vi "Perform Measurement.vi"(7 "error in (no error)":errorcluster, 8 "Measure Call Context in":refnum<class "Measure Call Context.lvclass">, 10 "measurement configuration":T2={"Mode of operation"=enum."Power on the DUT", "Source enable/disable"=FALSE, "Load enable/disable"=FALSE, "Source resource names"=[], "Load resource names"=[], "Power ON/Source system configuration"=enum."Series", "Power ON/Source output function"=0, "Source sweep scale"="", "Power ON V/I Source start level"=0.0, "Source stop level"=0.0, "Source sweep points/points per decade"=0, "Source voltage/current level range"=0.0, "Power ON/Source sense"=0, "Source limit symmetry"=enum."Symmetric", "Power ON/Source current/voltage limit range"=0.0, "Source current/voltage limit low"=0.0, "Source current/voltage limit high"=0.0, "Source source delay"=0.0, "Source aperture time"=0.0, "Source transient response"=0, "Source voltage/current gain bandwidth"=0.0, "Source voltage/current compensation frequency"=0.0, "Source voltage/current pole-zero ratio"=0.0, "Load system configuration"=enum."Series", "Load output function"=0, "Load device voltage/current rating"=50.0, "Load sweep scale"="", "Load start level"=0.0, "Load stop level"=0.0, "Load sweep points/points per decade"=0, "Load voltage/current level range"=0.0, "Load sense"=0, "Load limit symmetry"=enum."Symmetric", "Load current/voltage limit range"=0.0, "Load current/voltage limit low"=0.0, "Load current/voltage limit high"=0.0, "Load source delay"=0.0, "Load aperture time"=0.0, "Load transient response"=0, "Load voltage/current gain bandwidth"=0.0, "Load voltage/current compensation frequency"=0.0, "Load voltage/current pole-zero ratio"=0.0, "Load source trigger"="", "Load measure trigger"="", "Measurement timeout"=10.0} {"Measurement timeout" format="%.3p"; "Load device voltage/current rating" format="%#_6pA"; "Load output function" items=["DC Voltage"=1006, "DC Current"=1007, "Pulse Voltage"=1049, "Pulse Current"=1050]; "Power ON/Source output function" items=["DC Voltage"=1006, "DC Current"=1007, "Pulse Voltage"=1049, "Pulse Current"=1050]; "Load sweep points/points per decade" format="%#_6p"; "Power ON V/I Source start level" format="%#_6p"; "Load sense" items=["Symmetric", "Asymmetric"]; "Load transient response" items=["Slow"=1041, "Normal"=1038, "Fast"=1039, "Custom"=1042]; "Power ON/Source sense" items=["Local"=1008, "Remote"=1009]; "Source transient response" items=["Slow"=1041, "Normal"=1038, "Fast"=1039, "Custom"=1042]; "Load current/voltage limit low" format="%#_6p"; "Load current/voltage limit range" format="%#_6p"; "Load voltage/current level range" format="%#_6p"; "Source current/voltage limit high" format="%#_6p"; "Source current/voltage limit low" format="%#_6p"; "Power ON/Source current/voltage limit range" format="%#_6p"; "Source voltage/current level range" format="%#_6p"}) -> (0 "error out":errorcluster, 1 "Measure Call Context out":refnum<class "Measure Call Context.lvclass">, 3 "Measurement Results":T1)   [LabVIEW 2021, in "Sweep_Channel Ganging.lvlib"]
doc: "This VI Perform different API calls to do Sweep Measurement in different configurations of Source and Load like \n\nSingle-Ganged \nGanged-Ganged\nGanged-Single\nSingle-Single"
uses:
  Sweep_Channel Ganging.lvlib
  shared subVIs/ctl/NIDCPower_channel_ganging - ctl - ganged config.ctl
  shared subVIs/ctl/NIDCPower_channel_ganging - ctl - channel mode.ctl
  shared/Single/controls/Initialize Resource Config-Single.ctl
  shared/Ganging/controls/Initialize Resource Config-Ganging.ctl
  shared subVIs/ctl/NIDCPower_channel_ganging - ctl - ganged session.ctl
  <instrlib>/niDCPower/nidcpower.llb/niDCPower Wait For Event - Event.ctl
  Measurement Results.ctl
  ctl/Sweep fetch measurement control.ctl
  shared/Single/controls/Source to Sequence Config-Single.ctl
  shared/Ganging/controls/Source to Sequence Config-Ganging.ctl
  shared/Single/controls/Load to Sequence Config-Single.ctl
  shared/Ganging/controls/Load to Sequence Config-Ganging.ctl
  shared/Common/controls/Start and Wait for Event.ctl
  shared/Ganging/controls/Abort Single Point-Ganging.ctl
  shared/Single/controls/Abort Single Point-Single.ctl
  ctl/Sweep perform meaasurement.ctl
  <vilib>/Plug-In SDKs/Measurements/Measure Call Context/Measure Call Context.lvclass
  Measurement Configuration.ctl
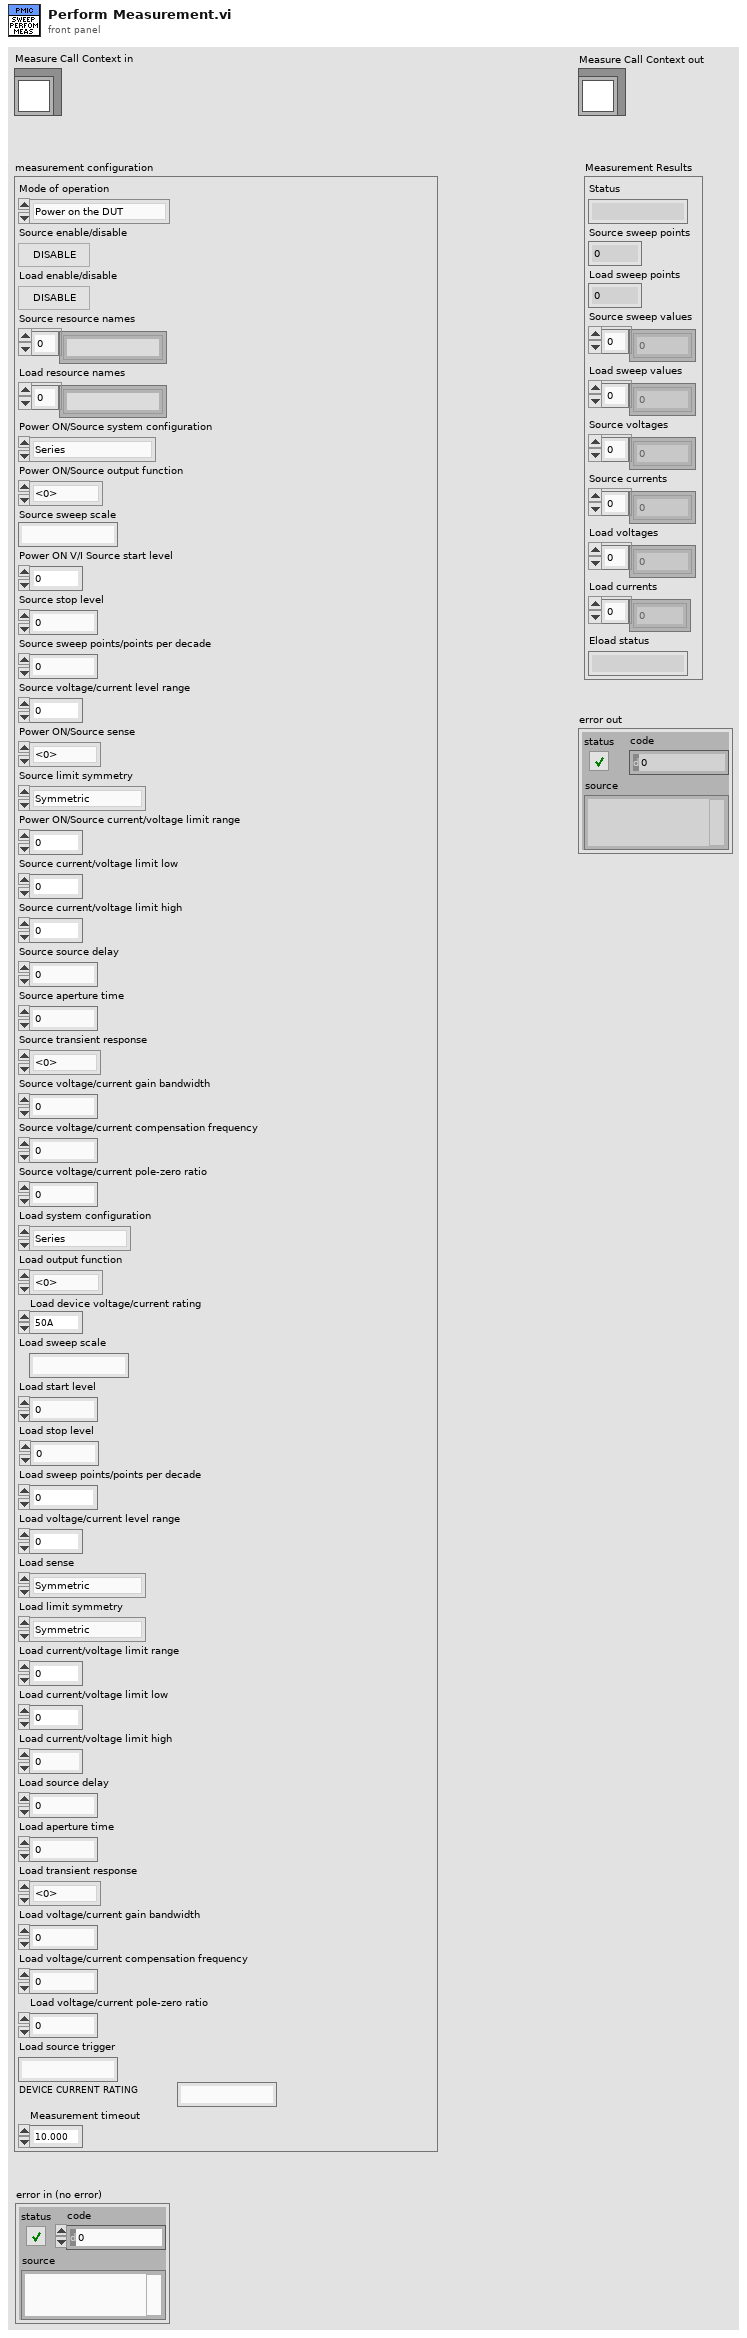
[diagram p1: front panel]
types:
  T1 = typedef "Sweep_Channel Ganging.lvlib/Measurement Results.ctl" = cluster{"Status":string, "Source sweep points":i32, "Load sweep points":i32, "Source sweep values":dbl[], "Load sweep values":dbl[], "Source voltages":dbl[], "Source currents":dbl[], "Load voltages":dbl[], "Load currents":dbl[], "Eload status":string}
  T2 = typedef "Sweep_Channel Ganging.lvlib/Measurement Configuration.ctl" = cluster{"Mode of operation":enum32{"Power on the DUT", "Perform measurement", "Power off the DUT"}, "Source enable/disable":bool, "Load enable/disable":bool, "Source resource names":string[], "Load resource names":string[], "Power ON/Source system configuration":enum32{"Series", "Parallel", "Manual"}, "Power ON/Source output function":i32, "Source sweep scale":string, "Power ON V/I Source start level":dbl, "Source stop level":dbl, "Source sweep points/points per decade":i32, "Source voltage/current level range":dbl, "Power ON/Source sense":i32, "Source limit symmetry":enum32{"Symmetric", "Asymmetric"}, "Power ON/Source current/voltage limit range":dbl, "Source current/voltage limit low":dbl, "Source current/voltage limit high":dbl, "Source source delay":dbl, "Source aperture time":dbl, "Source transient response":i32, "Source voltage/current gain bandwidth":dbl, "Source voltage/current compensation frequency":dbl, "Source voltage/current pole-zero ratio":dbl, "Load system configuration":enum32{"Series", "Parallel", "Manual"}, "Load output function":i32, "Load device voltage/current rating":dbl, "Load sweep scale":string, "Load start level":dbl, "Load stop level":dbl, "Load sweep points/points per decade":i32, "Load voltage/current level range":dbl, "Load sense":i32, "Load limit symmetry":enum32{"Symmetric", "Asymmetric"}, "Load current/voltage limit range":dbl, "Load current/voltage limit low":dbl, "Load current/voltage limit high":dbl, "Load source delay":dbl, "Load aperture time":dbl, "Load transient response":i32, "Load voltage/current gain bandwidth":dbl, "Load voltage/current compensation frequency":dbl, "Load voltage/current pole-zero ratio":dbl, "Load source trigger":string, "Load measure trigger":string, "Measurement timeout":dbl}
  T3 = typedef "Sweep_Channel Ganging.lvlib/Sweep perform meaasurement.ctl" = cluster{"Source Ganged Session Out":T4, "Load Ganged Session Out":T4, "Source sweep values":dbl[], "Source sweep points":i32, "Load sweep values":dbl[], "Load sweep points":i32, "Measurement Results":T1, "Source Master/Single resource name":string, "Source Slave resource name":string[], "Load Master/Single resource name":string, "Load Slave resource name":string[], "Load ganged/single":bool, "Source ganged/single":bool, "Source channel name":string, "Load channel name":string, "Source session out":refnum<k15>, "Load session out":refnum<k15>, "Number of Eload used":i32, "Load Source ON/OFF":enum16{"SOURCE AND LOAD OFF", "SOURCE ON", "LOAD ON", "SOURCE AND LOAD ON"}}
  T4 = typedef "NIDCPower_channel_ganging - ctl - ganged session.ctl" = cluster{"Ganged Config":T5, "Session List":refnum<k15>[], "Session Mode":T6[], "Channel":string[]}
  T5 = typedef "NIDCPower_channel_ganging - ctl - ganged config.ctl" = enum32{"Series", "Parallel", "Manual"}
  T6 = typedef "NIDCPower_channel_ganging - ctl - channel mode.ctl" = enum32{"Master", "Slave", "Slave - Inverted"}
  T7 = typedef "Initialize Resource Config-Single.ctl" = cluster{"Resource name":string, "Voltage/current level":dbl, "Voltage/current level range":dbl, "Voltage/current limit range":dbl, "Voltage/current limit low":dbl, "Voltage/current limit high":dbl, "Output function":i32, "Sense":i32, "Transient response":i32, "Voltage/current gain bandwidth":dbl, "Voltage/current compensation frequency":dbl, "Voltage/current pole-zero ratio":dbl, "DUT set-up time":dbl, "Limit symmetry":enum32{"Symmetric", "Asymmetric"}}
  T8 = typedef "Initialize Resource Config-Ganging.ctl" = cluster{"Master resource name ":string, "Slave resource names":string[], "System configuration":enum32{"Series", "Parallel", "Manual"}, "Voltage/current level":dbl, "Voltage/current level range":dbl, "Limit symmetry":enum32{"Symmetric", "Asymmetric"}, "Voltage/current limit range":dbl, "Voltage/current limit low":dbl, "Voltage/current limit high":dbl, "Output function":i32, "Sense":i32, "Transient response":i32, "Voltage/current gain bandwith":dbl, "Voltage/current compensation frequency":dbl, "Voltage/current pole-zero ratio":dbl, "DUT set-up time":dbl}
  T9 = typedef "Source to Sequence Config-Single.ctl" = cluster{"Source channel name":string, "Source out":refnum<k15>, "Source sweep values":dbl[], "Load sweep points":i32, "Source output function":i32, "Source transient response":i32, "Source voltage/current gain bandwidth":dbl, "Source voltage/current compensation frequency":dbl, "Source voltage/current pole-zero ratio":dbl, "Source aperture time":dbl, "Source source delay":dbl}
  T10 = typedef "Source to Sequence Config-Ganging.ctl" = cluster{"Source Ganged Session Out":cluster{"Ganged Config":T5, "Session List":refnum<k15>[], "Session Mode":T6[], "Channel":string[]}, "Source sweep values":dbl[], "Load sweep points":i32, "Source output function":i32, "Source transient response":i32, "Source voltage/current gain bandwidth":dbl, "Source voltage/current compensation frequency":dbl, "Source voltage/current pole-zero ratio":dbl, "Source aperture time":dbl, "Source source delay":dbl}
  T11 = typedef "Load to Sequence Config-Single.ctl" = cluster{"Load channel name":string, "Load out":refnum<k15>, "Load sweep values":dbl[], "Source sweep points":i32, "Load output function":i32, "Load transient response":i32, "Load voltage/current gain bandwidth":dbl, "Load voltage/current compensation frequency":dbl, "Load voltage/current pole-zero ratio":dbl, "Load aperture time":dbl, "Load source delay":dbl, "Load measure trigger":string, "Load source trigger":string}
  T12 = typedef "Load to Sequence Config-Ganging.ctl" = cluster{"Load Ganged Session Out":cluster{"Ganged Config":T5, "Session List":refnum<k15>[], "Session Mode":T6[], "Channel":string[]}, "Load sweep values":dbl[], "Source sweep points":i32, "Load output function":i32, "Load transient response":i32, "Load voltage/current gain bandwidth":dbl, "Load voltage/current compensation frequency":dbl, "Load voltage/current pole-zero ratio":dbl, "Load aperture time":dbl, "Load source delay":dbl, "Load measure trigger":string, "Load source trigger":string}
  T13 = typedef "Start and Wait for Event.ctl" = cluster{"Source Ganged Session Out":T4, "Load Ganged Session Out":T4, "Source session out":refnum<k15>, "Load session out":refnum<k15>, "event":T14, "Source channel name":string, "Load channel name":string, "Load Source ON/OFF":enum16{"SOURCE AND LOAD OFF", "SOURCE ON", "LOAD ON", "SOURCE AND LOAD ON"}, "Load ganged/single":bool, "Source ganged/single":bool}
  T14 = typedef "niDCPower Wait For Event - Event.ctl" = i32
  T15 = typedef "Sweep_Channel Ganging.lvlib/Sweep fetch measurement control.ctl" = cluster{"Source Ganged Session Out":T4, "Load Ganged Session Out":T4, "Source sweep values":dbl[], "Source sweep points":i32, "Load sweep values":dbl[], "Load sweep points":i32, "Measurement Results":T1, "Load ganged/single":bool, "Source ganged/single":bool, "Source channel name":string, "Load channel name":string, "Source session out":refnum<k15>, "Load session out":refnum<k15>, "Load Source ON/OFF":enum16{"SOURCE AND LOAD OFF", "SOURCE ON", "LOAD ON", "SOURCE AND LOAD ON"}, "Measurement timeout":dbl}
  T16 = typedef "Abort Single Point-Ganging.ctl" = cluster{"Ganged Session in":cluster{"Ganged Config":T5, "Session List":refnum<k15>[], "Session Mode":T6[], "Channel":string[]}}
  T17 = typedef "Abort Single Point-Single.ctl" = cluster{"Resource out":refnum<k15>, "Resource channel name":string}
  T18 = enum32{"Power on the DUT", "Perform measurement", "Power off the DUT"}
  T19 = enum16{"SOURCE AND LOAD OFF", "SOURCE ON", "LOAD ON", "SOURCE AND LOAD ON"}
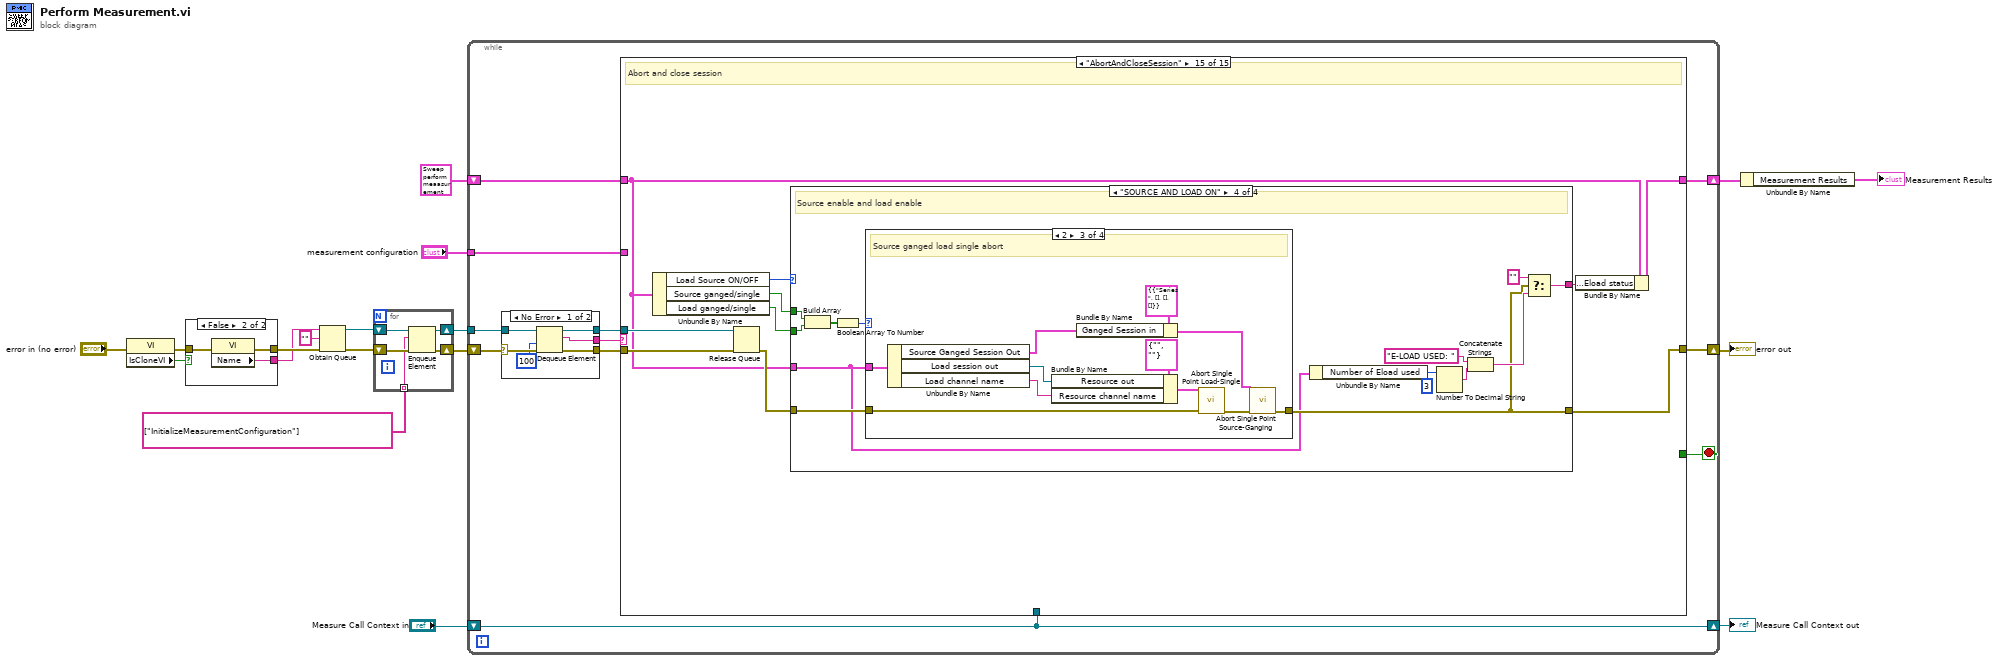
[diagram p0: block diagram]
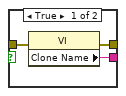
[diagram p2: hidden frame]
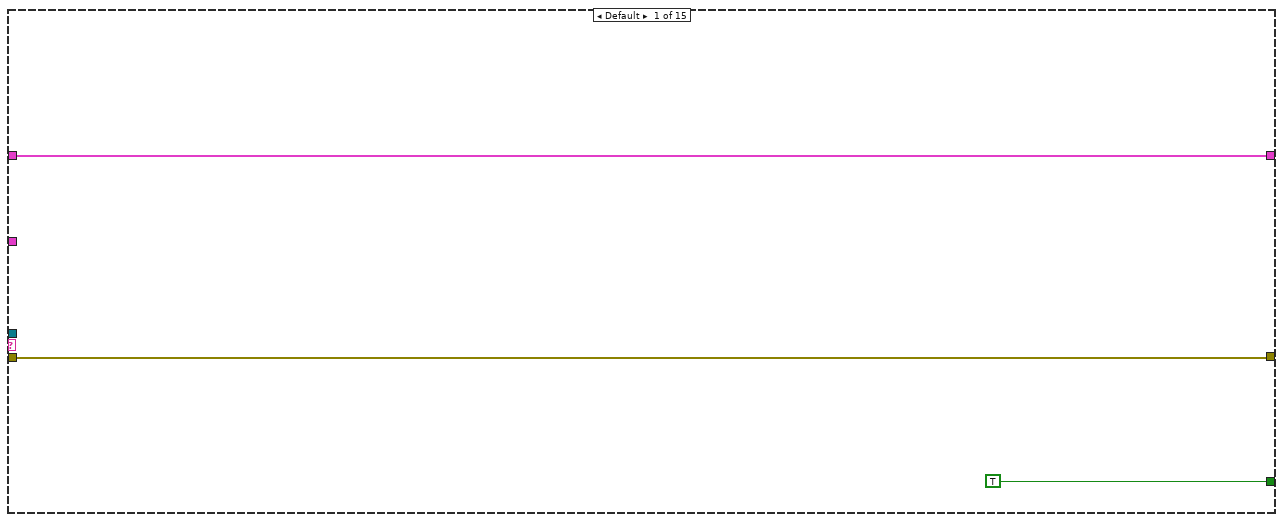
[diagram p3: hidden frame]
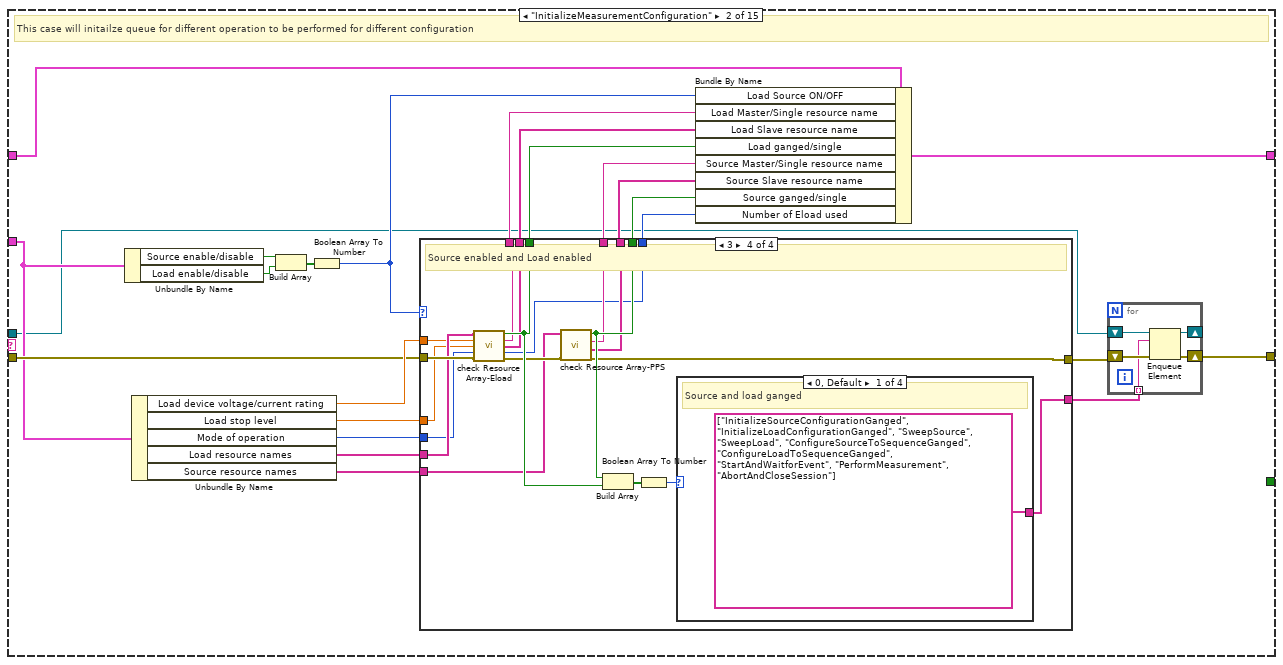
[diagram p4: hidden frame]
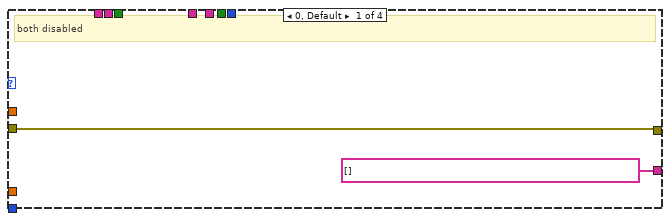
[diagram p5: hidden frame]
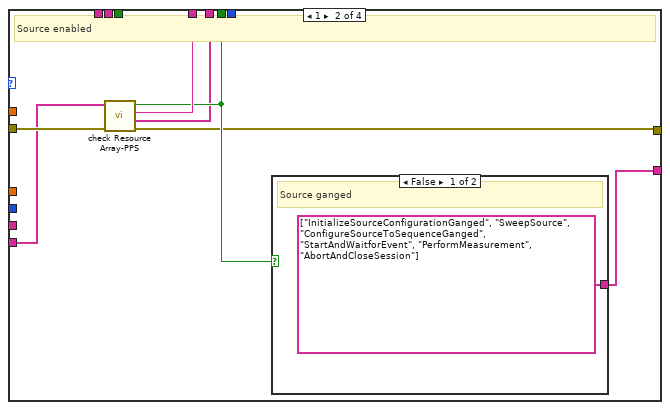
[diagram p6: hidden frame]
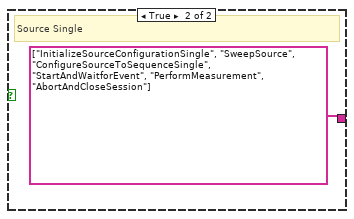
[diagram p7: hidden frame]
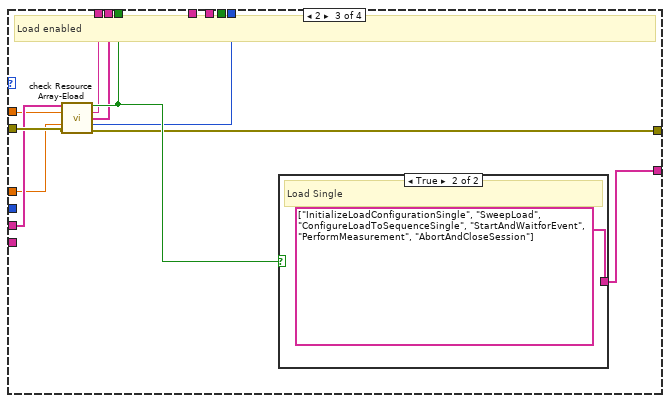
[diagram p8: hidden frame]
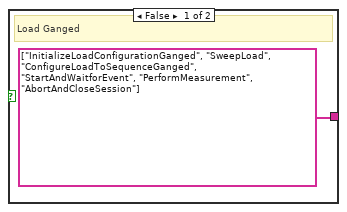
[diagram p9: hidden frame]
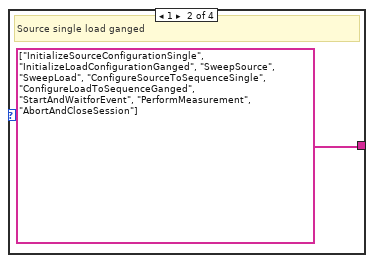
[diagram p10: hidden frame]
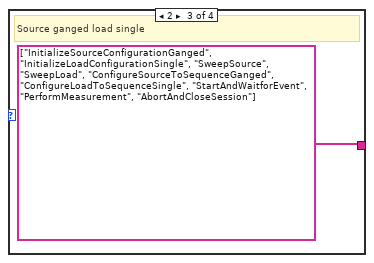
[diagram p11: hidden frame]
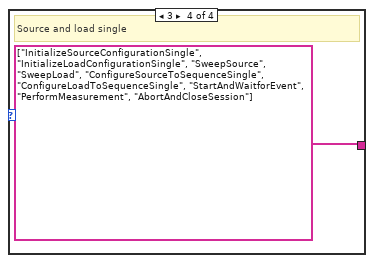
[diagram p12: hidden frame]
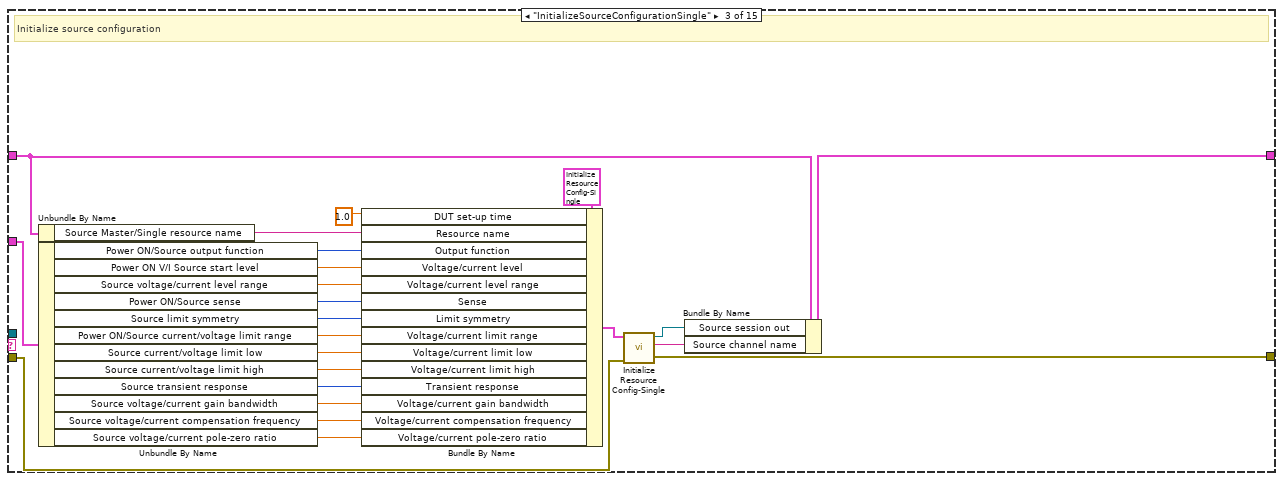
[diagram p13: hidden frame]
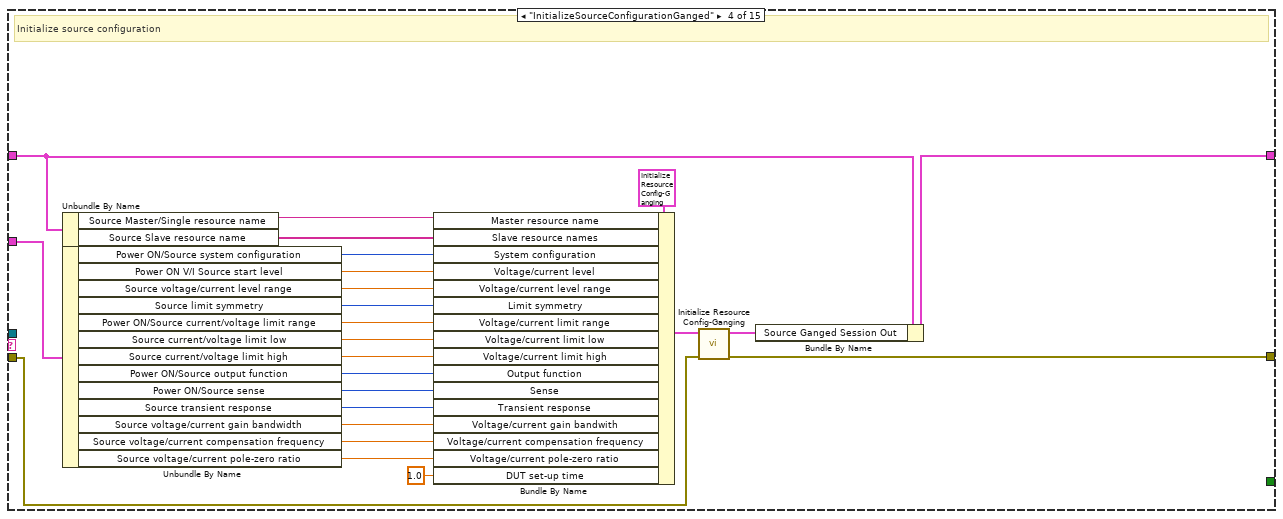
[diagram p14: hidden frame]
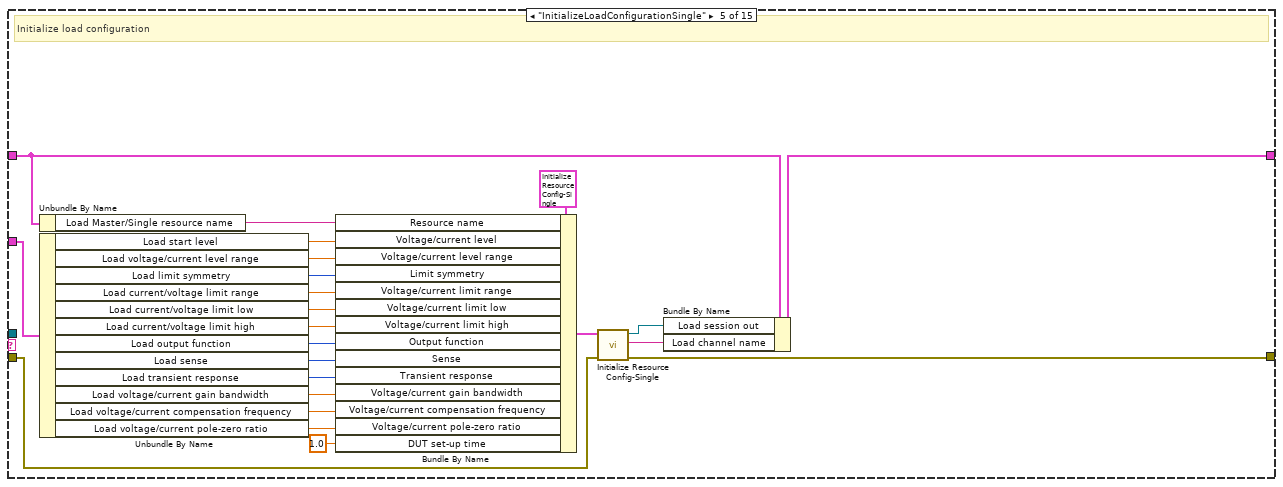
[diagram p15: hidden frame]
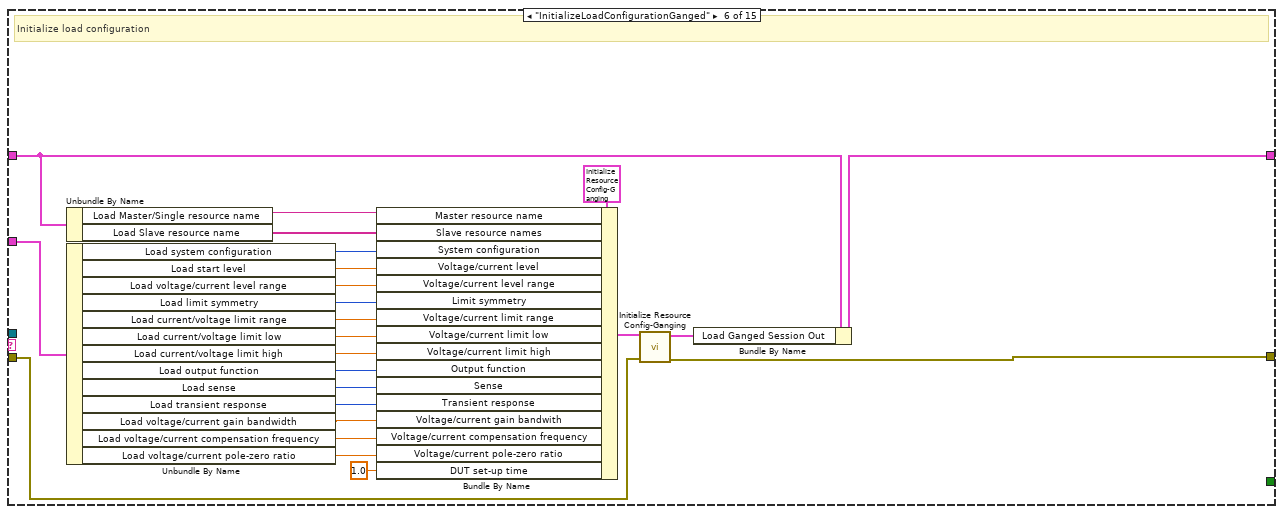
[diagram p16: hidden frame]
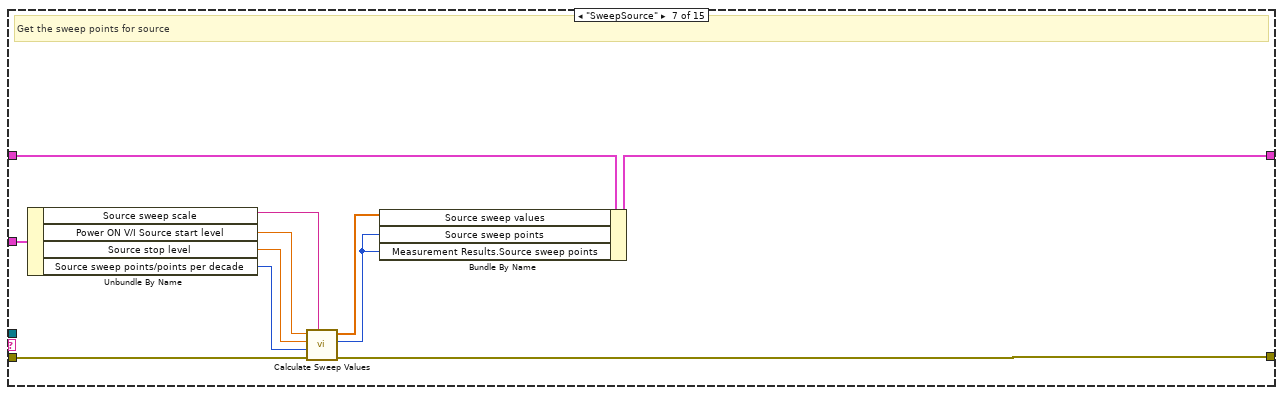
[diagram p17: hidden frame]
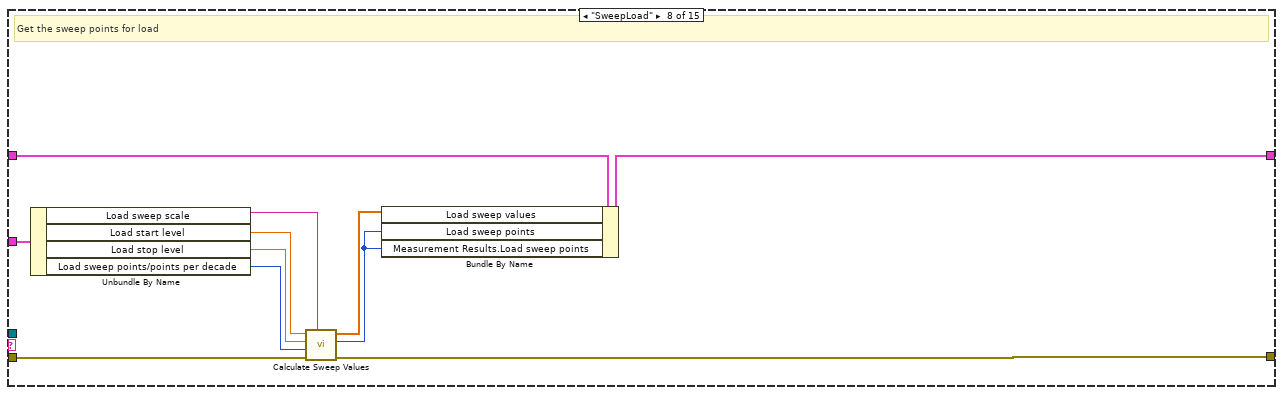
[diagram p18: hidden frame]
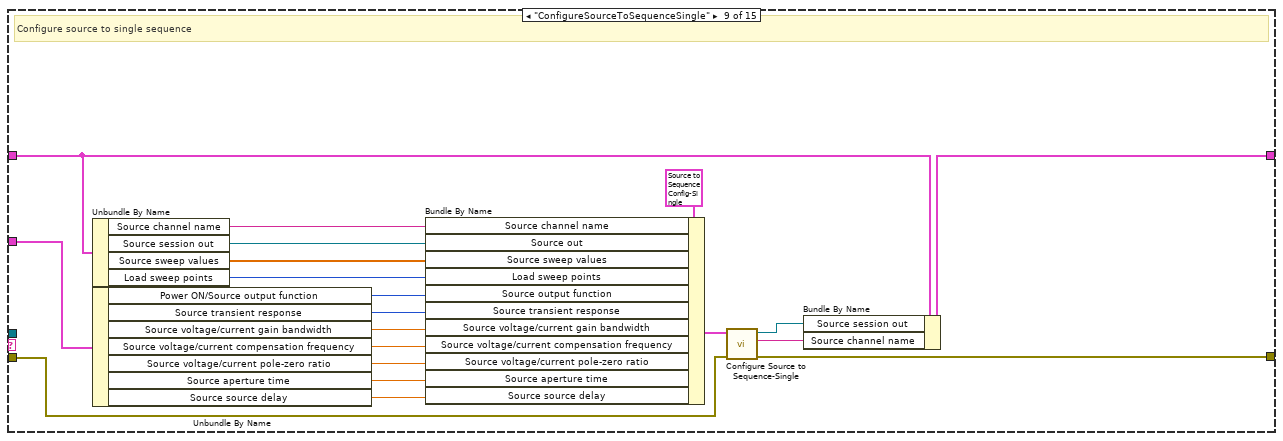
[diagram p19: hidden frame]
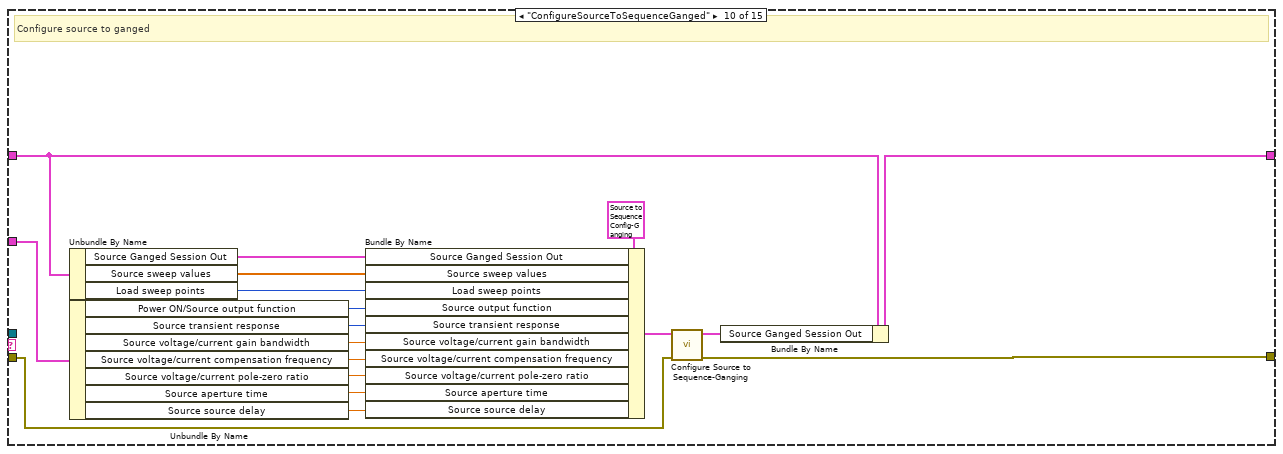
[diagram p20: hidden frame]
diagram:
  n1 = property class="VI"(error in="error in (no error)") -> (error out=w14:errorcluster, "IsCloneVI"=w13:bool)  [unwired: 1 in, 1 out]
  n2 = case shown="False" w13 {
    tunnel: [w21 w24] -> w6
    tunnel: [w20 w23] -> w4
    tunnel: w14 -> [w19 w22]
    frame True {
      n3 = property class="VI"(error in=w19) -> (error out=w21:errorcluster, "Clone Name"=w20:string)  [unwired: 1 in, 1 out]
    }
    frame False {
      n4 = property class="VI"(error in=w22) -> (error out=w24:errorcluster, "Name"=w23:string)  [unwired: 1 in, 1 out]
    }
  }
  n5 = Obtain Queue(name (unnamed)=w4, element data type="", error in (no error)=w6) -> (queue out=w9:refnum<queue>, error out=w10:errorcluster)  [unwired: 2 in, 1 out]
  n6 = for {
    shift-right: [w28] -> w5
    shift-left: w9 -> [w26]
    shift-right: [w27] -> w7
    shift-left: w10 -> [w29]
    tunnel: string[] ["InitializeMeasurementConfiguration"] ("Step sequence") -> [w25] mode=indexing
    n7 = Enqueue Element(queue=w26, element=w25, error in (no error)=w29) -> (queue out=w28:refnum<queue>, error out=w27:errorcluster)  [unwired: 1 in, 1 out]
  }
  n8 = while {
    shift-right: [w35] -> w2
    shift-left: T3 {"Source Ganged Session Out"={"Ganged Config"=enum."Series", "Session List"=[], "Session Mode"=[], "Channel"=[]}, "Load Ganged Session Out"={"Ganged Config"=enum."Series", "Session List"=[], "Session Mode"=[], "Channel"=[]}, "Source sweep values"=[], "Source sweep points"=0, "Load sweep values"=[], "Load sweep points"=0, "Measurement Results"={"Status"="", "Source sweep points"=0, "Load sweep points"=0, "Source sweep values"=[], "Load sweep values"=[], "Source voltages"=[], "Source currents"=[], "Load voltages"=[], "Load currents"=[], "Eload status"=""}, "Source Master/Single resource name"="", "Source Slave resource name"=[], "Load Master/Single resource name"="", "Load Slave resource name"=[], "Load ganged/single"=FALSE, "Source ganged/single"=FALSE, "Source channel name"="", "Load channel name"="", "Source session out"="", "Load session out"="", "Number of Eload used"=0, "Load Source ON/OFF"=enum."SOURCE AND LOAD OFF"} ("Sweep perform measurement control") -> [w36]
    shift-right: [w31] -> w17
    shift-left: w7 -> [w40]
    shift-right: [w34] -> w15
    shift-left: "Measure Call Context in" -> [w34]
    tunnel: "measurement configuration" -> [w32]
    tunnel: w5 -> [w30]
    stop <- w33 stop-if-true
    n9 = case shown="No Error" w40 {
      selector: w40 -> [w477 w480]
      tunnel: [w478 "Exit" ("t")] -> w39
      tunnel: [w476 w480] -> w37
      tunnel: [w474 w479] -> w38
      tunnel: w30 -> [w473 w479]
      frame No Error {
        n10 = Dequeue Element(queue=w473, timeout in ms (-1)=100, error in (no error)=w477) -> (queue out=w474:refnum<queue>, element=w478:string, error out=w476:errorcluster)  [unwired: 1 out]
      }
      frame Error {
      }
    }
    n11 = case shown="\"AbortAndCloseSession\"" w39 {
      tunnel: w38 -> [_ w45 _ _ _ _ _ _ _ _ _ _ _ _ w371]
      tunnel: w37 -> [w42 w51 w120 w146 w167 w207 w222 w233 w237 w257 w276 w297 w319 w342 w372]
      tunnel: w36 -> [w43 w52 w124 w144 w169 w206 w216 w227 w250 w268 w291 w311 w327 w357 w364]
      tunnel: [w43 w53 w123 w145 w168 w205 w213 w226 w251 w271 w293 w313 w326 w359 w363] -> w35
      tunnel: w34 -> [_ _ _ _ _ _ _ _ _ _ _ _ _ w340 _]
      tunnel: [TRUE _ _ _ _ _ _ _ _ _ _ _ _ _ TRUE] -> w33
      tunnel: w32 -> [_ w50 w140 w147 w185 w208 w221 w232 w249 w269 w290 w310 _ w338 _]
      tunnel: [w42 w48 w119 w142 w166 w189 w212 w224 w236 w256 w275 w296 w318 w361 w365] -> w31
      frame Default {
      }
      frame "InitializeMeasurementConfiguration" {
        # "This case will initailze queue for different operation to be performed for different configuration"
        n12 = Unbundle By Name(w50) -> ("Source enable/disable"=w56:bool, "Load enable/disable"=w55:bool)
        n13 = Unbundle By Name(w50) -> ("Load device voltage/current rating"=w66:dbl, "Load stop level"=w67:dbl, "Mode of operation"=w44:T18, "Load resource names"=w57:string[], "Source resource names"=w58:string[])
        n14 = Build Array(w56, w55) -> (w54:bool[])
        n15 = Boolean Array To Number(Boolean array=w54) -> (number=w59:u32)
        n16 = case shown="3" w59 {
          tunnel: w51 -> [w73 w81 w93 w111]
          tunnel: [w73 w76 w86 w100] -> w47
          tunnel: w57 -> [_ _ w92 w110]
          tunnel: w58 -> [_ w80 _ w102]
          tunnel: [_ _ w90 w108] -> w60
          tunnel: [_ _ w89 w107] -> w61
          tunnel: [_ w79 _ w104] -> w62
          tunnel: [_ w77 _ w103] -> w63
          tunnel: [_ _ w91 w109] -> w64
          tunnel: [_ w78 _ w105] -> w65
          tunnel: w66 -> [_ _ w88 w101]
          tunnel: w67 -> [_ _ w87 w97]
          tunnel: [string[] [] ("Step sequence") w75 w85 w98] -> w49
          tunnel: [_ _ w84 w99] -> w46
          tunnel: w44 -> [_ _ _ w96]
          frame 0, Default {
            # "both disabled"
          }
          frame 1 {
            # "Source enabled"
            n17 = call "check Resource Array-PPS.vi"("error in"=w81, "Resource names"=w80) -> ("error out"=w76:errorcluster, "Slave resource names"=w77:string[], "Single/Master resouce names"=w79:string, "Single or ganged configuration"=w78:bool)  [unwired: 6 in]
            n18 = case shown="False" w78 {
              tunnel: [string[] ["InitializeSourceConfigurationGanged", "SweepSource", "ConfigureSourceToSequenceGanged", "StartAndWaitforEvent", "PerformMeasurement", "AbortAndCloseSession"] ("Step sequence") string[] ["InitializeSourceConfigurationSingle", "SweepSource", "ConfigureSourceToSequenceSingle", "StartAndWaitforEvent", "PerformMeasurement", "AbortAndCloseSession"] ("Step sequence")] -> w75
              frame False {
                # "Source ganged"
              }
              frame True {
                # "Source Single"
              }
            }
          }
          frame 2 {
            # "Load enabled"
            n19 = call "check Resource Array-Eload.vi"("Resource names"=w92, "Device current rating"=w88, "Mode of operation"=w87, "error in"=w93) -> ("Single or ganged configuration"=w91:bool, "Single/Master resouce name"=w90:string, "Slave resource names"=w89:string[], "Number of devices used"=w84:i32, "error out"=w86:errorcluster)  [unwired: 7 in]
            n20 = case shown="True" w91 {
              tunnel: [string[] ["InitializeLoadConfigurationGanged", "SweepLoad", "ConfigureLoadToSequenceGanged", "StartAndWaitforEvent", "PerformMeasurement", "AbortAndCloseSession"] ("Step sequence") string[] ["InitializeLoadConfigurationSingle", "SweepLoad", "ConfigureLoadToSequenceSingle", "StartAndWaitforEvent", "PerformMeasurement", "AbortAndCloseSession"] ("Step sequence")] -> w85
              frame False {
                # "Load Ganged"
              }
              frame True {
                # "Load Single"
              }
            }
          }
          frame 3 {
            # "Source enabled and Load enabled"
            n21 = call "check Resource Array-Eload.vi"("Resource names"=w110, "Device current rating"=w101, "Expected current level"=w97, "Mode of operation"=w96, "error in"=w111) -> ("Single or ganged configuration"=w109:bool, "Single/Master resouce name"=w108:string, "Slave resource names"=w107:string[], "Number of devices used"=w99:i32, "error out"=w106:errorcluster)  [unwired: 6 in]
            n22 = call "check Resource Array-PPS.vi"("error in"=w106, "Resource names"=w102) -> ("error out"=w100:errorcluster, "Slave resource names"=w103:string[], "Single/Master resouce names"=w104:string, "Single or ganged configuration"=w105:bool)  [unwired: 6 in]
            n23 = Build Array(w105, w109) -> (w113:bool[])
            n24 = Boolean Array To Number(Boolean array=w113) -> (number=w112:u32)
            n25 = case shown="0, Default" w112 {
              tunnel: [string[] ["InitializeSourceConfigurationGanged", "InitializeLoadConfigurationGanged", "SweepSource", "SweepLoad", "ConfigureSourceToSequenceGanged", "ConfigureLoadToSequenceGanged", "StartAndWaitforEvent", "PerformMeasurement", "AbortAndCloseSession"] ("Step sequence") string[] ["InitializeSourceConfigurationSingle", "InitializeLoadConfigurationGanged", "SweepSource", "SweepLoad", "ConfigureSourceToSequenceSingle", "ConfigureLoadToSequenceGanged", "StartAndWaitforEvent", "PerformMeasurement", "AbortAndCloseSession"] ("Step sequence") string[] ["InitializeSourceConfigurationGanged", "InitializeLoadConfigurationSingle", "SweepSource", "SweepLoad", "ConfigureSourceToSequenceGanged", "ConfigureLoadToSequenceSingle", "StartAndWaitforEvent", "PerformMeasurement", "AbortAndCloseSession"] ("Step sequence") string[] ["InitializeSourceConfigurationSingle", "InitializeLoadConfigurationSingle", "SweepSource", "SweepLoad", "ConfigureSourceToSequenceSingle", "ConfigureLoadToSequenceSingle", "StartAndWaitforEvent", "PerformMeasurement", "AbortAndCloseSession"] ("Step sequence")] -> w98
              frame 0, Default {
                # "Source and load ganged"
              }
              frame 1 {
                # "Source single load ganged"
              }
              frame 2 {
                # "Source ganged load single"
              }
              frame 3 {
                # "Source and load single"
              }
            }
          }
        }
        n26 = Bundle By Name(cluster=w52, "Load Source ON/OFF"=w59, "Load Master/Single resource name"=w60, "Load Slave resource name"=w61, "Load ganged/single"=w64, "Source Master/Single resource name"=w62, "Source Slave resource name"=w63, "Source ganged/single"=w65, "Number of Eload used"=w46) -> (w53:T3)
        n27 = for {
          shift-right: [w70] -> _
          shift-left: w45 -> [w72]
          shift-right: [w69] -> w48
          shift-left: w47 -> [w71]
          tunnel: w49 -> [w68] mode=indexing
          n28 = Enqueue Element(queue=w72, element=w68, error in (no error)=w71) -> (queue out=w70:refnum<queue>, error out=w69:errorcluster)  [unwired: 1 in, 1 out]
        }
      }
      frame "InitializeSourceConfigurationSingle" {
        # "Initialize source configuration"
        n29 = Unbundle By Name(w124) -> ("Source Master/Single resource name"=w125:string)
        n30 = Unbundle By Name(w140) -> ("Power ON/Source output function"=w139:i32, "Power ON V/I Source start level"=w138:dbl, "Source voltage/current level range"=w137:dbl, "Power ON/Source sense"=w136:i32, "Source limit symmetry"=w135:enum32{"Symmetric", "Asymmetric"}, "Power ON/Source current/voltage limit range"=w134:dbl, "Source current/voltage limit low"=w133:dbl, "Source current/voltage limit high"=w132:dbl, "Source transient response"=w131:i32, "Source voltage/current gain bandwidth"=w130:dbl, "Source voltage/current compensation frequency"=w129:dbl, "Source voltage/current pole-zero ratio"=w128:dbl)
        n31 = Bundle By Name(cluster=T7 {"Resource name"="", "Voltage/current level"=0.0, "Voltage/current level range"=0.0, "Voltage/current limit range"=0.0, "Voltage/current limit low"=0.0, "Voltage/current limit high"=inf, "Output function"=1007, "Sense"=1009, "Transient response"=1038, "Voltage/current gain bandwidth"=0.0, "Voltage/current compensation frequency"=0.0, "Voltage/current pole-zero ratio"=0.0, "DUT set-up time"=0.0, "Limit symmetry"=enum."Symmetric"} ("Initialize Resource Config - Single"), "DUT set-up time"=1.0, "Resource name"=w125, "Output function"=w139, "Voltage/current level"=w138, "Voltage/current level range"=w137, "Sense"=w136, "Limit symmetry"=w135, "Voltage/current limit range"=w134, "Voltage/current limit low"=w133, "Voltage/current limit high"=w132, "Transient response"=w131, "Voltage/current gain bandwidth"=w130, "Voltage/current compensation frequency"=w129, "Voltage/current pole-zero ratio"=w128) -> (w126:T7)
        n32 = call "Initialize Resource Config-Single.vi"("error in"=w120, "Initialize resource Config - Single"=w126) -> ("error out"=w119:errorcluster, "channel name"=w122:string, "instrument handle out"=w121:refnum<k15>)  [unwired: 7 in]
        n33 = Bundle By Name(cluster=w124, "Source session out"=w121, "Source channel name"=w122) -> (w123:T3)
      }
      frame "InitializeSourceConfigurationGanged" {
        # "Initialize source configuration"
        n34 = Unbundle By Name(w144) -> ("Source Master/Single resource name"=w162:string, "Source Slave resource name"=w161:string[])
        n35 = Unbundle By Name(w147) -> ("Power ON/Source system configuration"=w160:enum32{"Series", "Parallel", "Manual"}, "Power ON V/I Source start level"=w159:dbl, "Source voltage/current level range"=w158:dbl, "Source limit symmetry"=w157:enum32{"Symmetric", "Asymmetric"}, "Power ON/Source current/voltage limit range"=w148:dbl, "Source current/voltage limit low"=w149:dbl, "Source current/voltage limit high"=w150:dbl, "Power ON/Source output function"=w151:i32, "Power ON/Source sense"=w152:i32, "Source transient response"=w153:i32, "Source voltage/current gain bandwidth"=w156:dbl, "Source voltage/current compensation frequency"=w155:dbl, "Source voltage/current pole-zero ratio"=w154:dbl)
        n36 = Bundle By Name(cluster=T8 {"Master resource name "="", "Slave resource names"=[], "System configuration"=enum."Parallel", "Voltage/current level"=0.0, "Voltage/current level range"=0.0, "Limit symmetry"=enum."Symmetric", "Voltage/current limit range"=0.0, "Voltage/current limit low"=0.0, "Voltage/current limit high"=inf, "Output function"=1007, "Sense"=1009, "Transient response"=1038, "Voltage/current gain bandwith"=0.0, "Voltage/current compensation frequency"=0.0, "Voltage/current pole-zero ratio"=0.0, "DUT set-up time"=0.0} ("Initialize Resource Config - Ganging"), "Master resource name"=w162, "Slave resource names"=w161, "System configuration"=w160, "Voltage/current level"=w159, "Voltage/current level range"=w158, "Limit symmetry"=w157, "Voltage/current limit range"=w148, "Voltage/current limit low"=w149, "Voltage/current limit high"=w150, "Output function"=w151, "Sense"=w152, "Transient response"=w153, "Voltage/current gain bandwith"=w156, "Voltage/current compensation frequency"=w155, "Voltage/current pole-zero ratio"=w154, "DUT set-up time"=1.0) -> (w164:T8)
        n37 = call "Initialize Resource Config-Ganging.vi"("error in"=w146, "Initialize Resource Config - Ganging"=w164) -> ("error out"=w142:errorcluster, "Ganged Session Out"=w143:T4)  [unwired: 8 in]
        n38 = Bundle By Name(cluster=w144, "Source Ganged Session Out"=w143) -> (w145:T3)
      }
      frame "InitializeLoadConfigurationSingle" {
        # "Initialize load configuration"
        n39 = Unbundle By Name(w169) -> ("Load Master/Single resource name"=w184:string)
        n40 = Unbundle By Name(w185) -> ("Load start level"=w172:dbl, "Load voltage/current level range"=w173:dbl, "Load limit symmetry"=w174:enum32{"Symmetric", "Asymmetric"}, "Load current/voltage limit range"=w175:dbl, "Load current/voltage limit low"=w176:dbl, "Load current/voltage limit high"=w177:dbl, "Load output function"=w178:i32, "Load sense"=w179:i32, "Load transient response"=w183:i32, "Load voltage/current gain bandwidth"=w182:dbl, "Load voltage/current compensation frequency"=w181:dbl, "Load voltage/current pole-zero ratio"=w180:dbl)
        n41 = Bundle By Name(cluster=T7 {"Resource name"="", "Voltage/current level"=0.0, "Voltage/current level range"=0.0, "Voltage/current limit range"=0.0, "Voltage/current limit low"=0.0, "Voltage/current limit high"=inf, "Output function"=1007, "Sense"=1009, "Transient response"=1038, "Voltage/current gain bandwidth"=0.0, "Voltage/current compensation frequency"=0.0, "Voltage/current pole-zero ratio"=0.0, "DUT set-up time"=0.0, "Limit symmetry"=enum."Symmetric"} ("Initialize Resource Config - Single"), "Resource name"=w184, "Voltage/current level"=w172, "Voltage/current level range"=w173, "Limit symmetry"=w174, "Voltage/current limit range"=w175, "Voltage/current limit low"=w176, "Voltage/current limit high"=w177, "Output function"=w178, "Sense"=w179, "Transient response"=w183, "Voltage/current gain bandwidth"=w182, "Voltage/current compensation frequency"=w181, "Voltage/current pole-zero ratio"=w180, "DUT set-up time"=1.0) -> (w186:T7)
        n42 = call "Initialize Resource Config-Single.vi"("error in"=w167, "Initialize resource Config - Single"=w186) -> ("error out"=w166:errorcluster, "channel name"=w170:string, "instrument handle out"=w171:refnum<k15>)  [unwired: 7 in]
        n43 = Bundle By Name(cluster=w169, "Load session out"=w171, "Load channel name"=w170) -> (w168:T3)
      }
      frame "InitializeLoadConfigurationGanged" {
        # "Initialize load configuration"
        n44 = Unbundle By Name(w206) -> ("Load Master/Single resource name"=w204:string, "Load Slave resource name"=w203:string[])
        n45 = Unbundle By Name(w208) -> ("Load system configuration"=w202:enum32{"Series", "Parallel", "Manual"}, "Load start level"=w201:dbl, "Load voltage/current level range"=w200:dbl, "Load limit symmetry"=w199:enum32{"Symmetric", "Asymmetric"}, "Load current/voltage limit range"=w198:dbl, "Load current/voltage limit low"=w197:dbl, "Load current/voltage limit high"=w196:dbl, "Load output function"=w195:i32, "Load sense"=w194:i32, "Load transient response"=w193:i32, "Load voltage/current gain bandwidth"=w192:dbl, "Load voltage/current compensation frequency"=w191:dbl, "Load voltage/current pole-zero ratio"=w190:dbl)
        n46 = Bundle By Name(cluster=T8 {"Master resource name "="", "Slave resource names"=[], "System configuration"=enum."Parallel", "Voltage/current level"=0.0, "Voltage/current level range"=0.0, "Limit symmetry"=enum."Symmetric", "Voltage/current limit range"=0.0, "Voltage/current limit low"=0.0, "Voltage/current limit high"=inf, "Output function"=1007, "Sense"=1009, "Transient response"=1038, "Voltage/current gain bandwith"=0.0, "Voltage/current compensation frequency"=0.0, "Voltage/current pole-zero ratio"=0.0, "DUT set-up time"=0.0} ("Initialize Resource Config - Ganging"), "Master resource name"=w204, "Slave resource names"=w203, "System configuration"=w202, "Voltage/current level"=w201, "Voltage/current level range"=w200, "Limit symmetry"=w199, "Voltage/current limit range"=w198, "Voltage/current limit low"=w197, "Voltage/current limit high"=w196, "Output function"=w195, "Sense"=w194, "Transient response"=w193, "Voltage/current gain bandwith"=w192, "Voltage/current compensation frequency"=w191, "Voltage/current pole-zero ratio"=w190, "DUT set-up time"=1.0) -> (w211:T8)
        n47 = call "Initialize Resource Config-Ganging.vi"("error in"=w207, "Initialize Resource Config - Ganging"=w211) -> ("error out"=w189:errorcluster, "Ganged Session Out"=w210:T4)  [unwired: 8 in]
        n48 = Bundle By Name(cluster=w206, "Load Ganged Session Out"=w210) -> (w205:T3)
      }
      frame "SweepSource" {
        # "Get the sweep points for source"
        n49 = Unbundle By Name(w221) -> ("Source sweep scale"=w220:string, "Power ON V/I Source start level"=w219:dbl, "Source stop level"=w218:dbl, "Source sweep points/points per decade"=w217:i32)
        n50 = call "Calculate Sweep Values.vi"("Sweep type"=w220, "error in"=w222, "Points"=w217, "Stop level"=w218, "Start level"=w219) -> ("error out"=w212:errorcluster, "Sweep points"=w214:i32, "Sweep values"=w215:dbl[])  [unwired: 4 in]
        n51 = Bundle By Name(cluster=w216, "Source sweep values"=w215, "Source sweep points"=w214, "Measurement Results.Source sweep points"=w214) -> (w213:T3)
      }
      frame "SweepLoad" {
        # "Get the sweep points for load"
        n52 = Unbundle By Name(w232) -> ("Load sweep scale"=w231:string, "Load start level"=w230:dbl, "Load stop level"=w229:dbl, "Load sweep points/points per decade"=w228:i32)
        n53 = call "Calculate Sweep Values.vi"("Sweep type"=w231, "error in"=w233, "Points"=w228, "Stop level"=w229, "Start level"=w230) -> ("error out"=w224:errorcluster, "Sweep points"=w225:i32, "Sweep values"=w223:dbl[])  [unwired: 4 in]
        n54 = Bundle By Name(cluster=w227, "Load sweep values"=w223, "Load sweep points"=w225, "Measurement Results.Load sweep points"=w225) -> (w226:T3)
      }
      frame "ConfigureSourceToSequenceSingle" {
        # "Configure source to single sequence"
        n55 = Unbundle By Name(w250) -> ("Source channel name"=w246:string, "Source session out"=w247:refnum<k15>, "Source sweep values"=w248:dbl[], "Load sweep points"=w245:i32)
        n56 = Unbundle By Name(w249) -> ("Power ON/Source output function"=w244:i32, "Source transient response"=w243:i32, "Source voltage/current gain bandwidth"=w242:dbl, "Source voltage/current compensation frequency"=w241:dbl, "Source voltage/current pole-zero ratio"=w240:dbl, "Source aperture time"=w239:dbl, "Source source delay"=w238:dbl)
        n57 = Bundle By Name(cluster=T9 {"Source channel name"="", "Source out"="", "Source sweep values"=[], "Load sweep points"=0, "Source output function"=1006, "Source transient response"=1038, "Source voltage/current gain bandwidth"=0.0, "Source voltage/current compensation frequency"=0.0, "Source voltage/current pole-zero ratio"=0.0, "Source aperture time"=0.0, "Source source delay"=0.0} ("Source to seq config - Single"), "Source channel name"=w246, "Source out"=w247, "Source sweep values"=w248, "Load sweep points"=w245, "Source output function"=w244, "Source transient response"=w243, "Source voltage/current gain bandwidth"=w242, "Source voltage/current compensation frequency"=w241, "Source voltage/current pole-zero ratio"=w240, "Source aperture time"=w239, "Source source delay"=w238) -> (w234:T9)
        n58 = call "Configure Source to Sequence-Single.vi"("error in"=w237, "Source to seq config - Single"=w234) -> ("error out"=w236:errorcluster, "Source channel name"=w252:string, "instrument handle out"=w253:refnum<k15>)  [unwired: 7 in]
        n59 = Bundle By Name(cluster=w250, "Source session out"=w253, "Source channel name"=w252) -> (w251:T3)
      }
      frame "ConfigureSourceToSequenceGanged" {
        # "Configure source to ganged"
        n60 = Unbundle By Name(w268) -> ("Source Ganged Session Out"=w260:T4, "Source sweep values"=w259:dbl[], "Load sweep points"=w258:i32)
        n61 = Unbundle By Name(w269) -> ("Power ON/Source output function"=w261:i32, "Source transient response"=w262:i32, "Source voltage/current gain bandwidth"=w263:dbl, "Source voltage/current compensation frequency"=w264:dbl, "Source voltage/current pole-zero ratio"=w265:dbl, "Source aperture time"=w266:dbl, "Source source delay"=w267:dbl)
        n62 = Bundle By Name(cluster=T10 {"Source Ganged Session Out"={"Ganged Config"=enum."Series", "Session List"=[], "Session Mode"=[], "Channel"=[]}, "Source sweep values"=[], "Load sweep points"=0, "Source output function"=1006, "Source transient response"=1038, "Source voltage/current gain bandwidth"=0.0, "Source voltage/current compensation frequency"=0.0, "Source voltage/current pole-zero ratio"=0.0, "Source aperture time"=0.0, "Source source delay"=0.0} ("Source to seq config - Ganging"), "Source Ganged Session Out"=w260, "Source sweep values"=w259, "Load sweep points"=w258, "Source output function"=w261, "Source transient response"=w262, "Source voltage/current gain bandwidth"=w263, "Source voltage/current compensation frequency"=w264, "Source voltage/current pole-zero ratio"=w265, "Source aperture time"=w266, "Source source delay"=w267) -> (w254:T10)
        n63 = call "Configure Source to Sequence-Ganging.vi"("error in"=w257, "Source to seq config - Ganging"=w254) -> ("error out"=w256:errorcluster, "Ganged Session Out"=w270:T4)  [unwired: 8 in]
        n64 = Bundle By Name(cluster=w268, "Source Ganged Session Out"=w270) -> (w271:T3)
      }
      frame "ConfigureLoadToSequenceSingle" {
        # "Configure load to single"
        n65 = Unbundle By Name(w291) -> ("Load channel name"=w289:string, "Load session out"=w288:refnum<k15>, "Load sweep values"=w287:dbl[], "Source sweep points"=w286:i32)
        n66 = Unbundle By Name(w290) -> ("Load output function"=w285:i32, "Load transient response"=w284:i32, "Load voltage/current gain bandwidth"=w283:dbl, "Load voltage/current compensation frequency"=w282:dbl, "Load voltage/current pole-zero ratio"=w281:dbl, "Load aperture time"=w280:dbl, "Load source delay"=w279:dbl, "Load measure trigger"=w278:string, "Load source trigger"=w277:string)
        n67 = Bundle By Name(cluster=T11 {"Load channel name"="", "Load out"="", "Load sweep values"=[], "Source sweep points"=0, "Load output function"=1007, "Load transient response"=1038, "Load voltage/current gain bandwidth"=0.0, "Load voltage/current compensation frequency"=0.0, "Load voltage/current pole-zero ratio"=0.0, "Load aperture time"=0.0, "Load source delay"=0.0, "Load measure trigger"="", "Load source trigger"=""} ("Load to seq config - Single"), "Load channel name"=w289, "Load out"=w288, "Load sweep values"=w287, "Source sweep points"=w286, "Load output function"=w285, "Load transient response"=w284, "Load voltage/current gain bandwidth"=w283, "Load voltage/current compensation frequency"=w282, "Load voltage/current pole-zero ratio"=w281, "Load aperture time"=w280, "Load source delay"=w279, "Load measure trigger"=w278, "Load source trigger"=w277) -> (w273:T11)
        n68 = call "Configure Load to Sequence-Single.vi"("error in"=w276, "Load to seq config - Single"=w273) -> ("error out"=w275:errorcluster, "Load channel Name"=w272:string, "instrument handle out"=w292:refnum<k15>)  [unwired: 7 in]
        n69 = Bundle By Name(cluster=w291, "Load session out"=w292, "Load channel name"=w272) -> (w293:T3)
      }
      frame "ConfigureLoadToSequenceGanged" {
        # "Configure load to ganged"
        n70 = Unbundle By Name(w311) -> ("Load Ganged Session Out"=w309:T4, "Load sweep values"=w308:dbl[], "Source sweep points"=w307:i32)
        n71 = Unbundle By Name(w310) -> ("Load output function"=w306:i32, "Load transient response"=w305:i32, "Load voltage/current gain bandwidth"=w304:dbl, "Load voltage/current compensation frequency"=w303:dbl, "Load voltage/current pole-zero ratio"=w302:dbl, "Load aperture time"=w301:dbl, "Load source delay"=w300:dbl, "Load measure trigger"=w299:string, "Load source trigger"=w298:string)
        n72 = Bundle By Name(cluster=T12 {"Load Ganged Session Out"={"Ganged Config"=enum."Series", "Session List"=[], "Session Mode"=[], "Channel"=[]}, "Load sweep values"=[], "Source sweep points"=0, "Load output function"=1007, "Load transient response"=1038, "Load voltage/current gain bandwidth"=0.0, "Load voltage/current compensation frequency"=0.0, "Load voltage/current pole-zero ratio"=0.0, "Load aperture time"=0.0, "Load source delay"=0.0, "Load measure trigger"="", "Load source trigger"=""} ("Load to seq config - Ganging"), "Load Ganged Session Out"=w309, "Load sweep values"=w308, "Source sweep points"=w307, "Load output function"=w306, "Load transient response"=w305, "Load voltage/current gain bandwidth"=w304, "Load voltage/current compensation frequency"=w303, "Load voltage/current pole-zero ratio"=w302, "Load aperture time"=w301, "Load source delay"=w300, "Load measure trigger"=w299, "Load source trigger"=w298) -> (w294:T12)
        n73 = call "Configure Load to Sequence-Ganging.vi"("error in"=w297, "Load to seq config - Ganging"=w294) -> ("error out"=w296:errorcluster, "Ganged Session Out"=w312:T4)  [unwired: 8 in]
        n74 = Bundle By Name(cluster=w311, "Load Ganged Session Out"=w312) -> (w313:T3)
      }
      frame "StartAndWaitforEvent" {
        w328 = T14 1033 items=["Source Complete Event"=1030, "Measure Complete Event"=1031, "Sequence Iteration Complete Event"=1032, "Sequence Engine Done Event"=1033, "Pulse Complete Event"=1051, "Ready For Pulse Trigger Event"=1052] ("event")
        # "Wait for event"
        n75 = Unbundle By Name(w327) -> ("Source Ganged Session Out"=w336:T4, "Load Ganged Session Out"=w335:T4, "Source session out"=w334:refnum<k15>, "Load session out"=w333:refnum<k15>, "Source channel name"=w332:string, "Load channel name"=w331:string, "Load Source ON/OFF"=w314:T19, "Load ganged/single"=w330:bool, "Source ganged/single"=w329:bool)
        n76 = Bundle By Name(cluster=T13 {"Source Ganged Session Out"={"Ganged Config"=enum."Series", "Session List"=[], "Session Mode"=[], "Channel"=[]}, "Load Ganged Session Out"={"Ganged Config"=enum."Series", "Session List"=[], "Session Mode"=[], "Channel"=[]}, "Source session out"="", "Load session out"="", "event"=1030, "Source channel name"="", "Load channel name"="", "Load Source ON/OFF"=enum."SOURCE AND LOAD OFF", "Load ganged/single"=FALSE, "Source ganged/single"=FALSE} ("Start and wait event config"), "Source Ganged Session Out"=w336, "Load Ganged Session Out"=w335, "Source session out"=w334, "Load session out"=w333, "Source channel name"=w332, "Load channel name"=w331, "Load Source ON/OFF"=w314, "Load ganged/single"=w330, "Source ganged/single"=w329, "event"=w328) -> (w315:T13)
        n77 = call "Start and Wait for Event.vi"("error in"=w319, "Start and wait event config"=w315) -> ("error out"=w318:errorcluster, "Start and wait event result"=w317:T13)  [unwired: 7 in]
        n78 = Unbundle By Name(w317) -> ("Source Ganged Session Out"=w325:T4, "Load Ganged Session Out"=w324:T4, "Source session out"=w323:refnum<k15>, "Load session out"=w322:refnum<k15>, "Source channel name"=w321:string, "Load channel name"=w320:string)
        n79 = Bundle By Name(cluster=w327, "Source Ganged Session Out"=w325, "Load Ganged Session Out"=w324, "Source session out"=w323, "Load session out"=w322, "Source channel name"=w321, "Load channel name"=w320) -> (w326:T3)
      }
      frame "PerformMeasurement" {
        # "Fetch Measurement"
        n80 = Unbundle By Name(w357) -> ("Load Source ON/OFF"=w356:T19, "Source Ganged Session Out"=w355:T4, "Load Ganged Session Out"=w354:T4, "Source sweep values"=w353:dbl[], "Source sweep points"=w352:i32, "Load sweep values"=w351:dbl[], "Load sweep points"=w350:i32, "Measurement Results"=w349:T1, "Load ganged/single"=w348:bool, "Source ganged/single"=w347:bool, "Source channel name"=w346:string, "Load channel name"=w345:string, "Source session out"=w344:refnum<k15>, "Load session out"=w343:refnum<k15>)
        n81 = Unbundle By Name(w338) -> ("Measurement timeout"=w337:dbl)
        n82 = Bundle By Name(cluster=T15 {"Source Ganged Session Out"={"Ganged Config"=enum."Series", "Session List"=[], "Session Mode"=[], "Channel"=[]}, "Load Ganged Session Out"={"Ganged Config"=enum."Series", "Session List"=[], "Session Mode"=[], "Channel"=[]}, "Source sweep values"=[], "Source sweep points"=0, "Load sweep values"=[], "Load sweep points"=0, "Measurement Results"={"Status"="", "Source sweep points"=0, "Load sweep points"=0, "Source sweep values"=[], "Load sweep values"=[], "Source voltages"=[], "Source currents"=[], "Load voltages"=[], "Load currents"=[], "Eload status"=""}, "Load ganged/single"=FALSE, "Source ganged/single"=FALSE, "Source channel name"="", "Load channel name"="", "Source session out"="", "Load session out"="", "Load Source ON/OFF"=enum."SOURCE AND LOAD OFF", "Measurement timeout"=10.0} ("Sweep fetch measurement control"), "Load Source ON/OFF"=w356, "Source Ganged Session Out"=w355, "Load Ganged Session Out"=w354, "Source sweep values"=w353, "Source sweep points"=w352, "Load sweep values"=w351, "Load sweep points"=w350, "Measurement Results"=w349, "Load ganged/single"=w348, "Source ganged/single"=w347, "Source channel name"=w346, "Load channel name"=w345, "Source session out"=w344, "Load session out"=w343, "Measurement timeout"=w337) -> (w339:T15)
        n83 = call "Fetch Measurement-Sweep.vi"("error in (no error)"=w342, "Measure Call Context in"=w340, "Sweep fetch measurement control"=w339) -> ("error out"=w361:errorcluster, "Sweep fetch measurement"=w341:T15)  [unwired: 7 in]
        n84 = Unbundle By Name(w341) -> ("Measurement Results"=w358:T1)
        n85 = Bundle By Name(cluster=w357, "Measurement Results"=w358) -> (w359:T3)
      }
      frame "AbortAndCloseSession" {
        # "Abort and close session"
        n86 = Unbundle By Name(w364) -> ("Load Source ON/OFF"=w369:T19, "Source ganged/single"=w367:bool, "Load ganged/single"=w368:bool)
        n87 = Release Queue(queue=w371, error in (no error)=w372) -> (error out=w366:errorcluster)  [unwired: 1 in, 2 out]
        n88 = case shown="\"SOURCE AND LOAD ON\"" w369 {
          tunnel: w367 -> [_ w379 _ w427]
          tunnel: w364 -> [_ w378 w393 w416]
          tunnel: w368 -> [_ _ w401 w428]
          tunnel: [w374 w377 w394 w417] -> w365
          tunnel: w366 -> [w374 w376 w402 w424]
          tunnel: ["" "" w395 w418] -> w362
          frame Default {
          }
          frame "SOURCE ON" {
            # "Source enable"
            n89 = case shown="True" w379 {
              tunnel: w378 -> [w385 w392]
              tunnel: [w381 w387] -> w377
              tunnel: w376 -> [w382 w388]
              frame False {
                # "Ganged channel abort"
                n90 = Unbundle By Name(w385) -> ("Source Ganged Session Out"=w383:T4)
                n91 = Bundle By Name(cluster=T16 {"Ganged Session in"={"Ganged Config"=enum."Series", "Session List"=[], "Session Mode"=[], "Channel"=[]}} ("Ganged Session Out"), "Ganged Session in"=w383) -> (w380:T16)
                n92 = call "Abort Single Point Source-Ganging.vi"("error in"=w382, "Ganged Session In"=w380) -> ("error out"=w381:errorcluster)  [unwired: 9 in]
              }
              frame True {
                # "Single channel abort"
                n93 = Unbundle By Name(w392) -> ("Source session out"=w391:refnum<k15>, "Source channel name"=w390:string)
                n94 = Bundle By Name(cluster=T17 {"Resource out"="", "Resource channel name"=""} ("Abort Single Point - Single"), "Resource out"=w391, "Resource channel name"=w390) -> (w386:T17)
                n95 = call "Abort Single Point Source-Single.vi"("error in"=w388, "Abort Single Point - Single"=w386) -> ("error out"=w387:errorcluster)  [unwired: 9 in]
              }
            }
          }
          frame "LOAD ON" {
            (unwired) i16 3 ("width (-)")
            # "Load enable"
            n96 = case shown="False" w401 {
              tunnel: w393 -> [w408 w415]
              tunnel: [w404 w410] -> w394
              tunnel: w402 -> [w405 w411]
              frame False {
                # "Ganged channel abort"
                n97 = Unbundle By Name(w408) -> ("Source Ganged Session Out"=w406:T4)
                n98 = Bundle By Name(cluster=T16 {"Ganged Session in"={"Ganged Config"=enum."Series", "Session List"=[], "Session Mode"=[], "Channel"=[]}} ("Ganged Session Out"), "Ganged Session in"=w406) -> (w403:T16)
                n99 = call "Abort Single Point Load-Ganging.vi"("error in"=w405, "Ganged Session In"=w403) -> ("error out"=w404:errorcluster)  [unwired: 9 in]
              }
              frame True {
                # "Single channel abort"
                n100 = Unbundle By Name(w415) -> ("Load session out"=w414:refnum<k15>, "Load channel name"=w413:string)
                n101 = Bundle By Name(cluster=T17 {"Resource out"="", "Resource channel name"=""} ("Abort Single Point - Single"), "Resource out"=w414, "Resource channel name"=w413) -> (w409:T17)
                n102 = call "Abort Single Point Load-Single.vi"("error in"=w411, "Abort Single Point - Single"=w409) -> ("error out"=w410:errorcluster)  [unwired: 9 in]
              }
            }
            n103 = Unbundle By Name(w393) -> ("Number of Eload used"=w399:i32)
            n104 = Number To Decimal String(number=w399) -> (decimal integer string=w400:string)  [unwired: 1 in]
            n105 = Concatenate Strings("E-LOAD USED: ", w400) -> (w397:string)
            n106 = Select(t="", s=w394, f=w397) -> (s? t:f=w395:string)
          }
          frame "SOURCE AND LOAD ON" {
            (unwired) i16 3 ("width (-)")
            # "Source enable and load enable"
            n107 = Build Array(w427, w428) -> (w426:bool[])
            n108 = Boolean Array To Number(Boolean array=w426) -> (number=w425:u32)
            n109 = case shown="2" w425 {
              tunnel: w416 -> [w438 w449 w460 w470]
              tunnel: [w433 w441 w452 w462] -> w417
              tunnel: w424 -> [w431 w443 w454 w464]
              frame 0, Default {
                # "Source and load ganged abort"
                n110 = Unbundle By Name(w438) -> ("Source Ganged Session Out"=w436:T4, "Load Ganged Session Out"=w437:T4)
                n111 = Bundle By Name(cluster=T16 {"Ganged Session in"={"Ganged Config"=enum."Series", "Session List"=[], "Session Mode"=[], "Channel"=[]}} ("Ganged Session In"), "Ganged Session in"=w436) -> (w429:T16)
                n112 = Bundle By Name(cluster=T16 {"Ganged Session in"={"Ganged Config"=enum."Series", "Session List"=[], "Session Mode"=[], "Channel"=[]}} ("Ganged Session In"), "Ganged Session in"=w437) -> (w430:T16)
                n113 = call "Abort Single Point Load-Ganging.vi"("error in"=w431, "Ganged Session In"=w430) -> ("error out"=w432:errorcluster)  [unwired: 9 in]
                n114 = call "Abort Single Point Source-Ganging.vi"("error in"=w432, "Ganged Session In"=w429) -> ("error out"=w433:errorcluster)  [unwired: 9 in]
              }
              frame 1 {
                # "Source single load ganged abort"
                n115 = Unbundle By Name(w449) -> ("Source session out"=w447:refnum<k15>, "Source channel name"=w446:string, "Load Ganged Session Out"=w448:T4)
                n116 = Bundle By Name(cluster=T17 {"Resource out"="", "Resource channel name"=""} ("Abort Single Point - Single"), "Resource out"=w447, "Resource channel name"=w446) -> (w440:T17)
                n117 = Bundle By Name(cluster=T16 {"Ganged Session in"={"Ganged Config"=enum."Series", "Session List"=[], "Session Mode"=[], "Channel"=[]}} ("Ganged Session In"), "Ganged Session in"=w448) -> (w439:T16)
                n118 = call "Abort Single Point Load-Ganging.vi"("error in"=w443, "Ganged Session In"=w439) -> ("error out"=w442:errorcluster)  [unwired: 9 in]
                n119 = call "Abort Single Point Source-Single.vi"("error in"=w442, "Abort Single Point - Single"=w440) -> ("error out"=w441:errorcluster)  [unwired: 9 in]
              }
              frame 2 {
                # "Source ganged load single abort"
                n120 = Unbundle By Name(w460) -> ("Source Ganged Session Out"=w457:T4, "Load session out"=w459:refnum<k15>, "Load channel name"=w458:string)
                n121 = Bundle By Name(cluster=T17 {"Resource out"="", "Resource channel name"=""} ("Abort Single Point - Single"), "Resource out"=w459, "Resource channel name"=w458) -> (w450:T17)
                n122 = Bundle By Name(cluster=T16 {"Ganged Session in"={"Ganged Config"=enum."Series", "Session List"=[], "Session Mode"=[], "Channel"=[]}} ("Ganged Session In"), "Ganged Session in"=w457) -> (w451:T16)
                n123 = call "Abort Single Point Load-Single.vi"("error in"=w454, "Abort Single Point - Single"=w450) -> ("error out"=w453:errorcluster)  [unwired: 9 in]
                n124 = call "Abort Single Point Source-Ganging.vi"("error in"=w453, "Ganged Session In"=w451) -> ("error out"=w452:errorcluster)  [unwired: 9 in]
              }
              frame 3 {
                # "Source and load single abort"
                n125 = Unbundle By Name(w470) -> ("Source session out"=w468:refnum<k15>, "Source channel name"=w469:string, "Load session out"=w472:refnum<k15>, "Load channel name"=w471:string)
                n126 = Bundle By Name(cluster=T17 {"Resource out"="", "Resource channel name"=""} ("Abort Single Point - Single"), "Resource out"=w468, "Resource channel name"=w469) -> (w461:T17)
                n127 = Bundle By Name(cluster=T17 {"Resource out"="", "Resource channel name"=""} ("Abort Single Point - Single"), "Resource out"=w472, "Resource channel name"=w471) -> (w465:T17)
                n128 = call "Abort Single Point Load-Single.vi"("error in"=w464, "Abort Single Point - Single"=w465) -> ("error out"=w463:errorcluster)  [unwired: 9 in]
                n129 = call "Abort Single Point Source-Single.vi"("error in"=w463, "Abort Single Point - Single"=w461) -> ("error out"=w462:errorcluster)  [unwired: 9 in]
              }
            }
            n130 = Unbundle By Name(w416) -> ("Number of Eload used"=w422:i32)
            n131 = Number To Decimal String(number=w422) -> (decimal integer string=w423:string)  [unwired: 1 in]
            n132 = Concatenate Strings("E-LOAD USED: ", w423) -> (w420:string)
            n133 = Select(t="", s=w417, f=w420) -> (s? t:f=w418:string)
          }
        }
        n134 = Bundle By Name(cluster=w364, "Measurement Results.Eload status"=w362) -> (w363:T3)
      }
    }
  }
  "error out" <- w17
  "Measure Call Context out" <- w15
  n135 = Unbundle By Name(w2) -> ("Measurement Results"=→"Measurement Results":T1)
